vi "Plugin.UDP.Get Connection ID.vi"(10 "id":i32, 11 "UDP Plugin in":refnum<class "UDP Plugin.lvclass">) -> (2 "connection ID":refnum<k16>, 3 "UDP Plugin out":refnum<class "UDP Plugin.lvclass">)   [LabVIEW 2017, in "UDP Plugin.lvclass"]
uses:
  UDP Plugin.lvclass
  UDP Plugin.lvclass/UDP Plugin.ctl
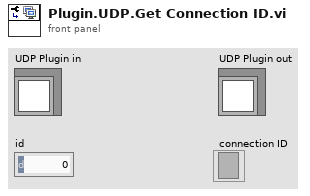
[diagram p1: front panel]
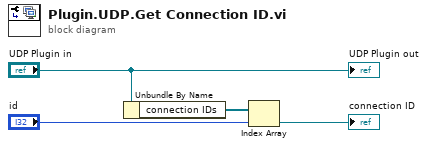
[diagram p0: block diagram]
diagram:
  n1 = Unbundle By Name("UDP Plugin in") -> ("connection IDs"=w3:refnum<k16>[])
  n2 = Index Array(array=w3, index="id") -> (element=→"connection ID":refnum<k16>)
  "UDP Plugin out" <- "UDP Plugin in"
